vi "Decrypt with AES.vi"(0 "Password.In":string, 2 "BitKeyType(256)":u16(ring)=256 items=["AES bit key 128"=128, "AES bit key 192"=192, "AES bit key 256"=256], 7 "Encrypted Text In":string, 11 "error in":errorcluster) -> (8 "Decrypted Text Out":string, 15 "error out":errorcluster)   [LabVIEW 2012, in "Advanced Encryption Standard (AES).lvlib"]
doc: "Takes string encrypted with Advanced Encryption Standart (AES) and decrypts it into initial text. \n\nThis VI allows reentrant execution."
uses:
  Advanced Encryption Standard (AES).lvlib
  Controls and Typedefs/Decryption Phases Enum (Typedef).ctl
  Controls and Typedefs/Decipher Phases Enum (Typedef).ctl
panel:
  out "unsigned byte.utf8":u8[](array[numeric])
  out "unsigned byte.text":u8[](array[numeric])
  out "plaintxtByte":i32[](array[numeric])
  out "ciphertextArr":string[](array[string])
  out "ct":string[](array[string])
  out "nBlocks":i32
  out "cipherCntr":u16[](array[numeric])
  in  "0x100000000":u64=4294967296 format="%.0x"
  in  "blockSize":i32=16
  out "keySchedule":u32[](array[numeric])
  out "ctrTxt":string
  out "counterBlock":u32[](array[numeric])
  out "pwBytes":u32[](array[numeric])
  out "nBytes":i32
  # "Number of bits used in the key (256 by default).\nThe longer a key, the higher level of protection\nat expence of processor and RAM usage."
  # "Advanced Encryption Standart (AES)\nAES Decrypt 1.0"
  # "Receives Password in String format (plain text)"
  # "Receives encrypted text needed to be decrypted"
  # "Decrypted (plain) text"
  # "Development and Debugging"
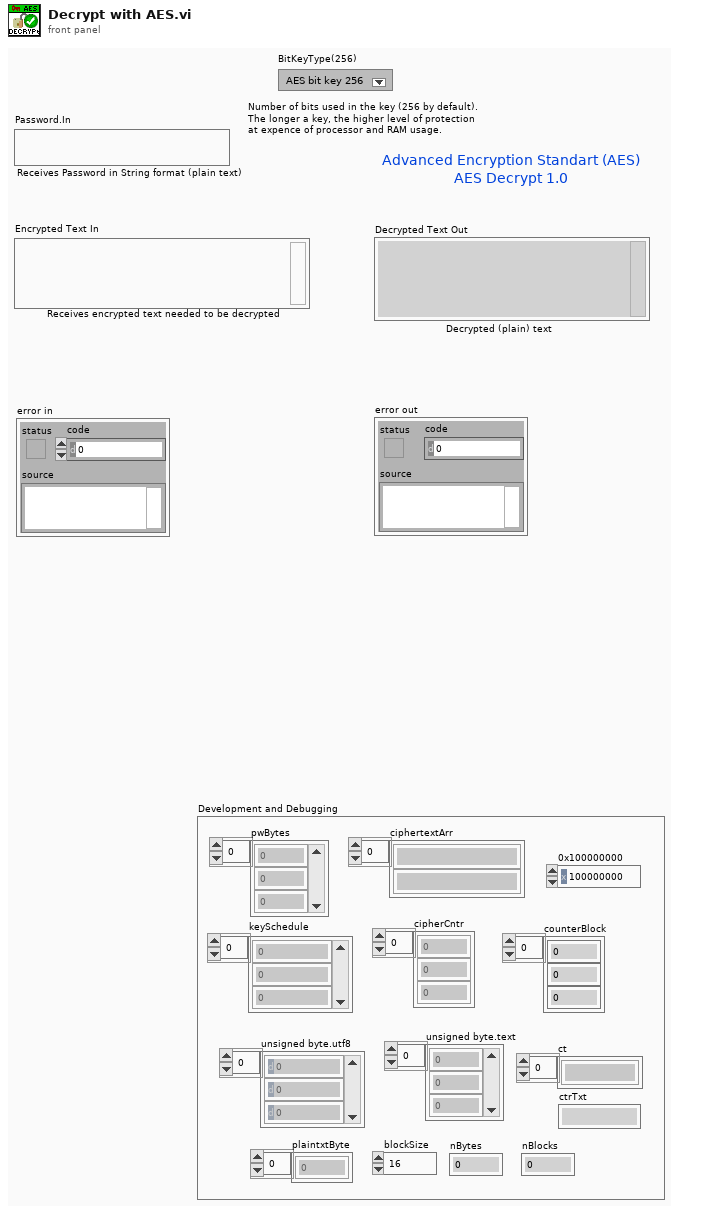
[diagram p1: front panel]
types:
  T1 = typedef "Decryption Phases Enum (Typedef).ctl" = enum16{"Init", "Decipher"}
  T2 = typedef "Decipher Phases Enum (Typedef).ctl" = enum16{"Logical Shifts", "Combine Bytes"}
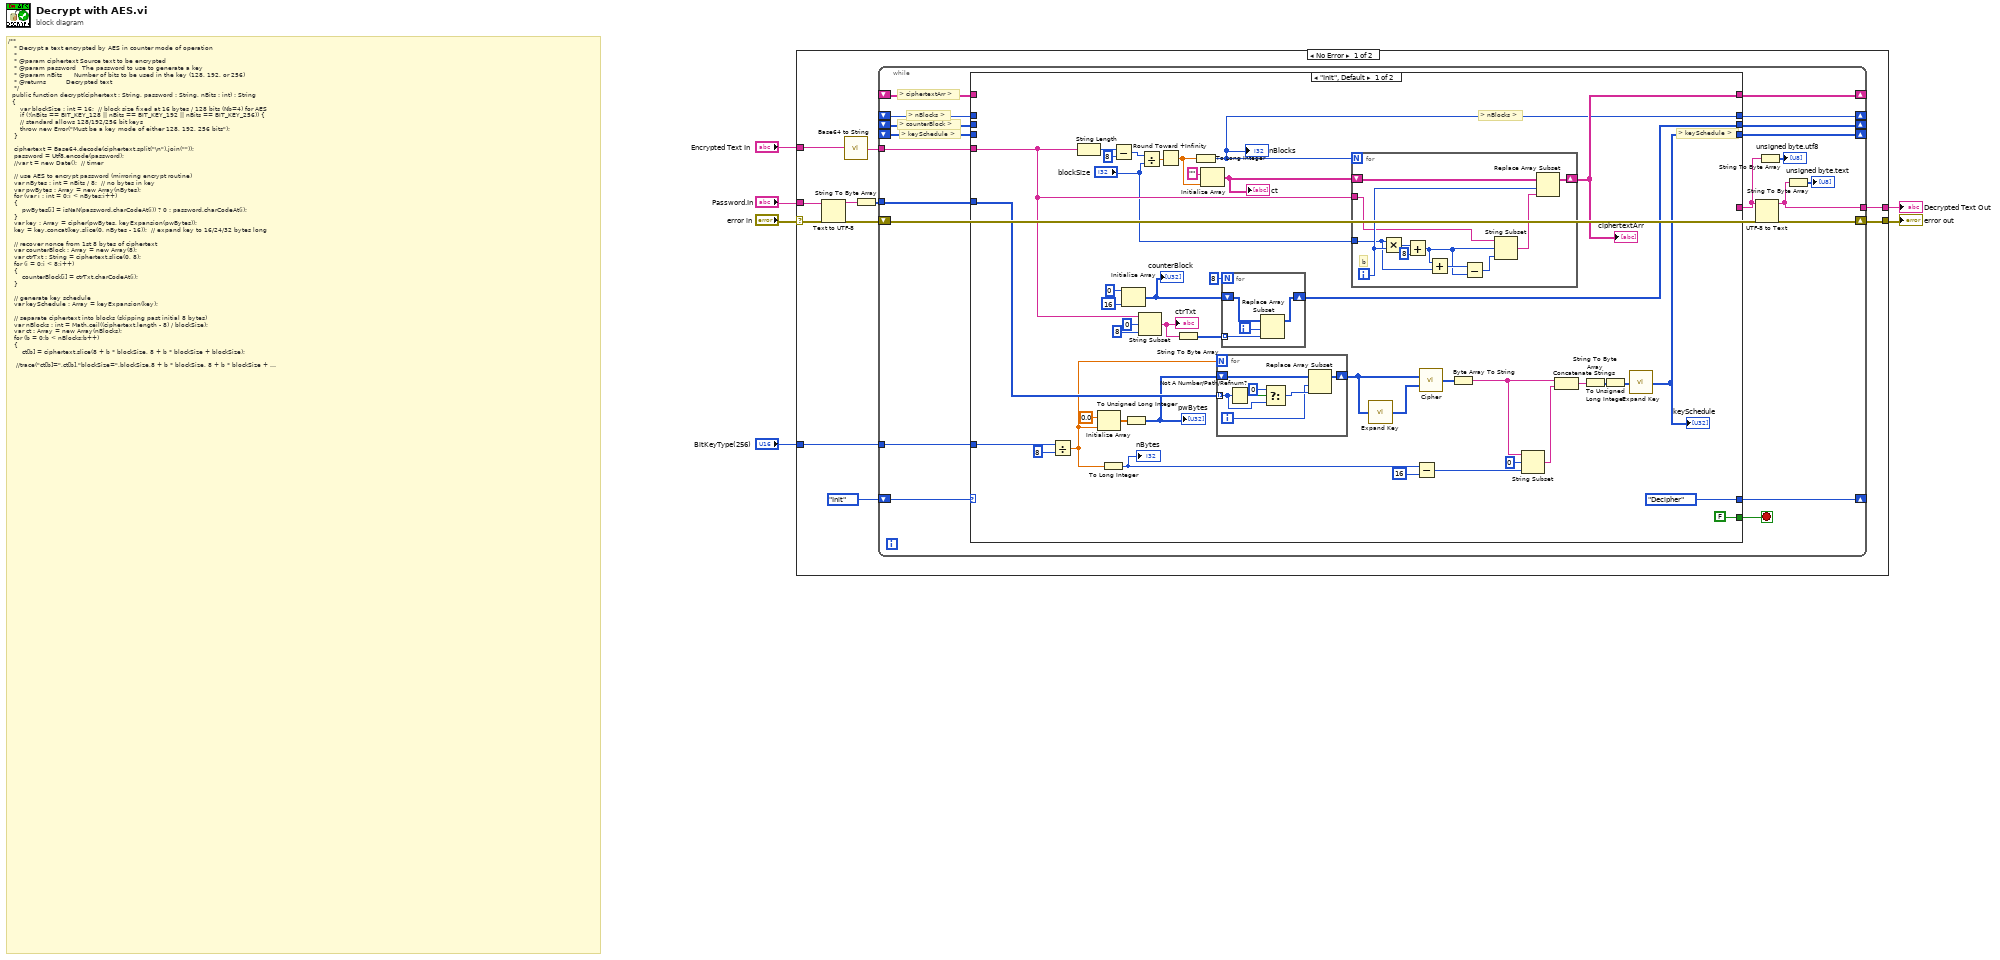
[diagram p0: block diagram]
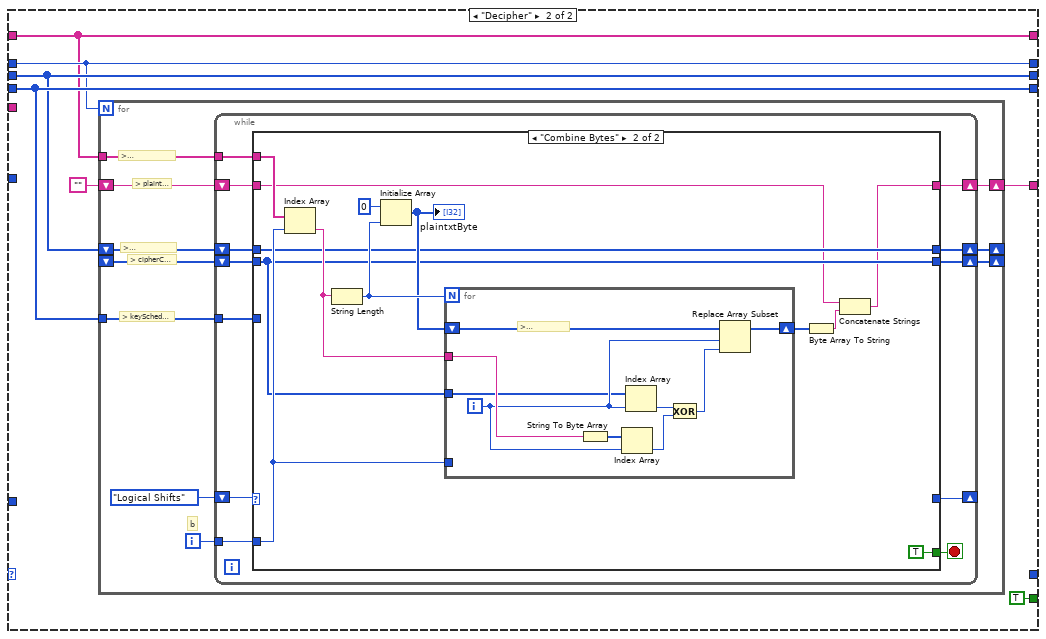
[diagram p2: hidden frame]
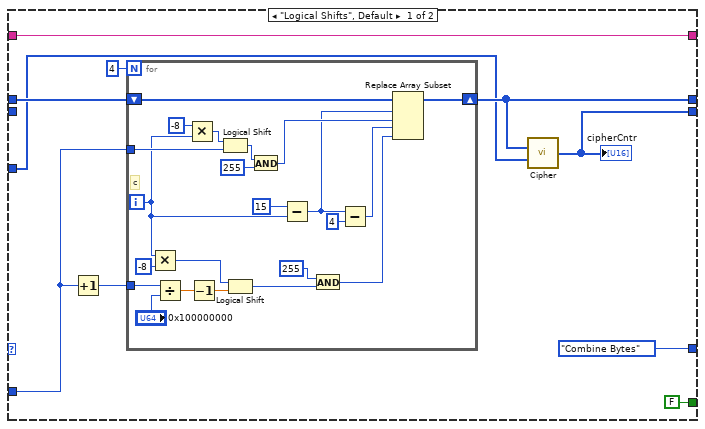
[diagram p3: hidden frame]
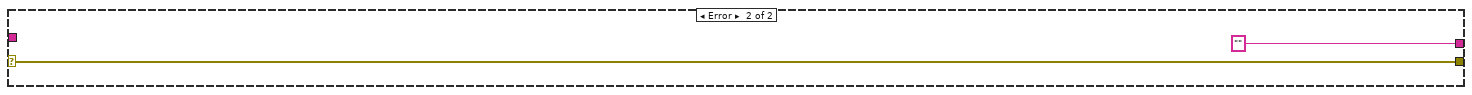
[diagram p4: hidden frame]
diagram:
  # "/** \n\t\t * Decrypt a text encrypted by AES in counter mode of operation\n\t\t *\n\t\t * @param ciphertext Source text to be encrypted\n\t\t * @param password   The password to use to generate a key\n\t\t * @param nBits      Number of bits to be used in the key (128, 192, or 256)\n\t\t * @returns          Decrypted text\n\t\t */\n\t\tpublic function decrypt(ciphertext : String, password : String, nBits : int) : String \n  {\n\t\t   \tvar blockSize : int = 16;  // block size fixed at 16 bytes / 128 bits (Nb=4) for AES\n\t\t   \tif (!(nBits == BIT_KEY_128 || nBits == BIT_KEY_192 || nBits == BIT_KEY_256)) {\n\t\t\t\t  // standard allows 128/192/256 bit keys\n\t\t\t\t  throw new Error(\"Must be a key mode of either 128, 192, 256 bits\");\n\t\t\t}\n\t\t\t\n\t\t\tciphertext = Base64.decode(ciphertext.split(\"\\n\").join(\"\"));\n\t\t\tpassword = Utf8.encode(password);\n\t\t\t//var t = new Date();  // timer\n\t\t\t  \n\t\t\t// use AES to encrypt password (mirroring encrypt routine)\n\t\t\tvar nBytes : int = nBits / 8;  // no bytes in key\n\t\t\tvar pwBytes : Array = new Array(nBytes);\n\t\t\tfor (var i : int = 0;i < nBytes;i++) \n\t\t\t{\n\t\t   \t\tpwBytes[i] = isNaN(password.charCodeAt(i)) ? 0 : password.charCodeAt(i);\n\t\t\t}\n\t\t\tvar key : Array = cipher(pwBytes, keyExpansion(pwBytes));\n\t\t\tkey = key.concat(key.slice(0, nBytes - 16));  // expand key to 16/24/32 bytes long\n\t\t\t\n\t\t\t// recover nonce from 1st 8 bytes of ciphertext\n\t\t\tvar counterBlock : Array = new Array(8);\n\t\t\tvar ctrTxt : String = ciphertext.slice(0, 8);\n\t\t\tfor (i = 0;i < 8;i++) \n\t\t\t{\n\t\t\t   \tcounterBlock[i] = ctrTxt.charCodeAt(i);\n\t\t\t}\n\t\t\t  \n\t\t\t// generate key schedule\n\t\t\tvar keySchedule : Array = keyExpansion(key);\n\t\t\t\n\t\t\t// separate ciphertext into blocks (skipping past initial 8 bytes)\n\t\t\tvar nBlocks : int = Math.ceil((ciphertext.length - 8) / blockSize);\n\t\t\tvar ct : Array = new Array(nBlocks);\n\t\t\tfor (b = 0;b < nBlocks;b++) \n\t\t\t{\n\t\t\t   \tct[b] = ciphertext.slice(8 + b * blockSize, 8 + b * blockSize + blockSize);\n\t\t\t\t\n\t\t\t\t//trace(\"ct[b]=\",ct[b],\"blockSize=\",blockSize,8 + b * blockSize, 8 + b * blockSize + blockSize);\n\t\t\t}\n\t\t\t//var temp:String=ct[1];\n//\t\t\tfor (var i:int=0;i<temp.length;i++)\n//\t\t\t{\n//\t\t\t\ttrace(\"ct[1]Byte Array:\",temp.charCodeAt(i));\n//\t\t\t}\n\t\t\t\n\t\t\tvar ciphertextArr : Array = ct;  // ciphertext is now array of block-length strings\n\t\t\t\n\t\t\t// plaintext will get generated block-by-block into array of block-length strings\n\t\t\tvar plaintxt : Array = new Array(ciphertextArr.length);\n\t\t\t\n\t\t\tfor (var b : int = 0;b < nBlocks;b++) \n\t\t\t{\n\t\t\t\t// set counter (block #) in last 8 bytes of counter block (leaving nonce in 1st 8 bytes)\n\t\t\t   \tfor (var c : int = 0;c < 4;c++) \n\t\t\t\t   {\n\t\t\t      \t\tcounterBlock[15 - c] = ((b) >>> c * 8) & 0xff;\n\t\t   \t\t}\n\t   \t\t\tfor (c = 0;c < 4;c++) \n\t  \t\t\t{\n\t\t     \t\t\tcounterBlock[15 - c - 4] = (((b + 1) / 0x100000000 - 1) >>> c * 8) & 0xff;\n\t\t\t  \t}\n\t\t\t\t//trace(counterBlock);\n\t\t\t\tvar cipherCntr : Array = cipher(counterBlock, keySchedule);  // encrypt counter block\n\t\t\t\t//trace(cipherCntr);\n\t\t\t\tvar plaintxtByte : Array = new Array(String(ciphertextArr[b]).length);\n\t\t\t\tfor (i = 0;i < String(ciphertextArr[b]).length;i++) \n\t\t\t\t{\n\t\t\t\t   \t// -- xor plaintxt with ciphered counter byte-by-byte --\n\t\t\t\t   \tplaintxtByte[i] = cipherCntr[i] ^ String(ciphertextArr[b]).charCodeAt(i);\n\t\t\t  \t\t//trace(\"i=\",i,\"plaintxtByte[i]=\",plaintxtByte[i],\"cipherCntr[i]=\",cipherCntr[i],\"String(ciphertextArr[b]).charCodeAt(i)=\",String(ciphertextArr[b]).charCodeAt(i));\n\t\t\t  \t\t//trace(plaintxtByte[i]);\n\t\t\t  \t\tplaintxtByte[i] = String.fromCharCode(plaintxtByte[i]);\n\t\t\t\t\t\n\t\t\t\t}\n\t\t\t\tplaintxt[b] = plaintxtByte.join('');\n\t\t\t}\n\t\t\t\n\t\t\t// join array of blocks into single plaintext string\n\t\t\tvar plaintext : String = plaintxt.join('');\n\t\t\tplaintext = Utf8.decode(plaintext);  // decode from UTF8 back to Unicode multi-byte chars\n\t\t\treturn plaintext;\n\t\t}"
  n1 = case shown="No Error" "error in" {
    selector: "error in" -> [w8 w186]
    tunnel: [w13 w186] -> w5
    tunnel: "Encrypted Text In" -> [w11 _]
    tunnel: "Password.In" -> [w10 _]
    tunnel: [w9 "" ("text")] -> w2
    tunnel: "BitKeyType(256)" -> [w7 _]
    frame No Error {
      n2 = Text to UTF-8(8:w8, 11:w10) -> (0:w12:errorcluster, 3:w16:string)
      n3 = call "Base64 to String.vi"("Base64 String"=w11) -> ("String"=w14:string)  [unwired: 13 in, 1 out]
      n4 = String To Byte Array(string=w16) -> (unsigned byte array=w15:u8[])
      n5 = while {
        shift-right: [w25] -> _
        shift-left: Decryption_Phases_Enum_(Typedef)."Init" ("Decrypt Phases") -> [w37]
        tunnel: w15 -> [w36]
        tunnel: w14 -> [w35]
        shift-right: [w33] -> _
        shift-left: _ -> [w32]
        shift-right: [w31] -> _
        shift-left: _ -> [w30]
        shift-right: [w29] -> _
        shift-left: _ -> [w28]
        shift-right: [w27] -> _
        shift-left: _ -> [w26]
        tunnel: [w21] -> w9
        shift-right: [w20] -> w13
        shift-left: w12 -> [w19]
        tunnel: w7 -> [w18]
        stop <- w34 stop-if-true
        # "> keySchedule >"
        # "> counterBlock >"
        # "> nBlocks >"
        # "> ciphertextArr >"
        n6 = case shown="\"Init\", Default" w37 {
          tunnel: w36 -> [w65 _]
          tunnel: w35 -> [w47 _]
          tunnel: [FALSE TRUE] -> w34
          tunnel: [w46 w104] -> w33
          tunnel: w32 -> [_ w104]
          tunnel: [w44 w105] -> w31
          tunnel: w30 -> [_ w105]
          tunnel: [w43 w106] -> w29
          tunnel: w28 -> [_ w106]
          tunnel: [w42 w108] -> w27
          tunnel: w26 -> [_ w108]
          tunnel: [Decryption_Phases_Enum_(Typedef)."Decipher" ("Decrypt Phases") _] -> w25
          tunnel: [_ w103] -> w22
          tunnel: w18 -> [w38 _]
          frame "Init", Default {
            # "> keySchedule >"
            # "> nBlocks >"
            n7 = Divide(x=w38, y=u16 8) -> (x/y=w52:dbl)
            n8 = String Length(string=w47) -> (length=w74:i32)
            n9 = Initialize Array(0.0 ("element"), w52) -> (w64:dbl[])
            n10 = To Long Integer(number=w52) -> (32bit integer=w51:i32)
            "nBytes" <- w51
            n11 = Subtract(x=w74, y=8) -> (x-y=w72:i32)
            n12 = Initialize Array(u32 0 ("y"), 16 ("dimension size")) -> (w62:u32[])
            "counterBlock" <- w62
            n13 = To Unsigned Long Integer(number=w64) -> (unsigned 32bit integer=w63:u32[])
            "pwBytes" <- w63
            n14 = String Subset(string=w47, offset (0)=0, length (rest)=8 ("length (rest)")) -> (substring=w68:string)
            "ctrTxt" <- w68
            n15 = Divide(x=w72, y="blockSize") -> (x/y=w71:dbl)
            n16 = Round Toward +Infinity(x=w71) -> (ceil(x): smallest int >= x=w50:dbl)
            n17 = String To Byte Array(string=w68) -> (unsigned byte array=w69:u8[])
            n18 = To Long Integer(number=w50) -> (32bit integer=w44:i32)
            "nBlocks" <- w44
            n19 = Initialize Array("", w50) -> (w49:string[])
            "ct" <- w49
            n20 = for {
              N: w52 -> [_]
              tunnel: w65 -> [w97] mode=indexing
              shift-right: [w95] -> w53
              shift-left: w63 -> [w96]
              i -> [w99]
              n21 = Not A Number/Path/Refnum?(number/path/refnum=w97) -> (NaN/Path/Refnum?=w101:bool)
              n22 = Select(t=0 ("f"), s=w101, f=w97) -> (s? t:f=w100:i32)
              n23 = Replace Array Subset(array=w96, new element=w100, index=w99) -> (w95:u32[])
            }
            n24 = for {
              N: 8 -> [_]
              tunnel: w69 -> [w94] mode=indexing
              shift-right: [w91] -> w43
              shift-left: w62 -> [w92]
              i -> [w93]
              n25 = Replace Array Subset(array=w92, new element=w94, index=w93) -> (w91:u32[])
            }
            n26 = for {
              N: w44 -> [_]
              shift-right: [w82] -> w46
              shift-left: w49 -> [w83]
              tunnel: w47 -> [w81]
              tunnel: "blockSize" -> [w80]
              i -> [w88]
              # "b"
              n27 = Multiply(x=w80, y=w88) -> (x*y=w90:i32)
              n28 = Add(x=w90, y=8) -> (x+y=w85:i32)
              n29 = Add(x=w85, y=w80) -> (x+y=w86:i32)
              n30 = Subtract(x=w86, y=w85) -> (x-y=w84:i32)
              n31 = String Subset(string=w81, offset (0)=w85, length (rest)=w84) -> (substring=w87:string)
              n32 = Replace Array Subset(array=w83, new element=w87, index=w88) -> (w82:string[])
            }
            "ciphertextArr" <- w46
            n33 = call "Expand Key.vi"("Key"=w53) -> ("Expanded Key"=w54:u32[])  [unwired: 13 in, 1 out]
            n34 = Subtract(x=w51, y=u8 16) -> (x-y=w59:i32)
            n35 = call "Cipher.vi"("Key(input)"=w53, "ExpandedKey(w)1D"=w54) -> ("Cypher Output"=w55:u16[])  [unwired: 12 in, 1 out]
            n36 = Byte Array To String(unsigned byte array=w55) -> (string=w56:string)
            n37 = String Subset(string=w56, offset (0)=0, length (rest)=w59) -> (substring=w60:string)
            n38 = Concatenate Strings(w56, w60) -> (w61:string)
            n39 = String To Byte Array(string=w61) -> (unsigned byte array=w41:u8[])
            n40 = To Unsigned Long Integer(number=w41) -> (unsigned 32bit integer=w40:u32[])
            n41 = call "Expand Key.vi"("Key"=w40) -> ("Expanded Key"=w42:u32[])  [unwired: 13 in, 1 out]
            "keySchedule" <- w42
          }
          frame "Decipher" {
            n42 = for {
              N: w105 -> [_]
              shift-right: [w116] -> _
              shift-left: w106 -> [w117]
              tunnel: w108 -> [w115]
              shift-right: [w114] -> _
              shift-left: _ -> [w113]
              tunnel: w104 -> [w112]
              shift-right: [w111] -> w103
              shift-left: "" -> [w110]
              i -> [w118]
              # "> keySchedule >"
              # "> ciphertextArr >"
              # "> plaintxt >"
              # "> cipherCntr >"
              # "> counterBlock >"
              # "b"
              n43 = while {
                tunnel: w118 -> [w130]
                shift-right: [w119] -> _
                shift-left: Decipher_Phases_Enum_(Typedef)."Logical Shifts" ("Decipher Phases") -> [w121]
                shift-right: [w128] -> w116
                shift-left: w117 -> [w129]
                tunnel: w115 -> [w127]
                shift-right: [w126] -> w114
                shift-left: w113 -> [w124]
                tunnel: w112 -> [w125]
                shift-right: [w123] -> w111
                shift-left: w110 -> [w122]
                stop <- w120 stop-if-true
                n44 = case shown="\"Combine Bytes\"" w121 {
                  tunnel: w130 -> [w138 w170]
                  tunnel: w129 -> [w137 w166]
                  tunnel: [w136 w166] -> w128
                  tunnel: w127 -> [w135 _]
                  tunnel: [w134 w167] -> w126
                  tunnel: w125 -> [_ w169]
                  tunnel: w124 -> [_ w167]
                  tunnel: [w133 w165] -> w123
                  tunnel: w122 -> [w133 w164]
                  tunnel: [FALSE TRUE] -> w120
                  tunnel: [Decipher_Phases_Enum_(Typedef)."Combine Bytes" ("Decipher Phases") _] -> w119
                  frame "Logical Shifts", Default {
                    n45 = Increment(x=w138) -> (x+1=w140:i32)
                    n46 = for {
                      N: 4 -> [_]
                      tunnel: w138 -> [w160]
                      tunnel: w140 -> [w154]
                      shift-right: [w141] -> w136
                      shift-left: w137 -> [w142]
                      i -> [w149]
                      # "c"
                      n47 = Multiply(x=w149, y=-8 ("x")) -> (x*y=w148:i32)
                      n48 = Divide(x=w154, y="0x100000000") -> (x/y=w151:dbl)
                      n49 = Multiply(x=-8, y=w149) -> (x*y=w153:i32)
                      n50 = Decrement(x=w151) -> (x-1=w147:dbl)
                      n51 = Logical Shift(y=w153, x=w160) -> (x << y=w162:i32)
                      n52 = Logical Shift(y=w148, x=w147) -> (x << y=w146:u32)
                      n53 = And(x=w162, y=u16 255 ("0xff")) -> (x .and. y?=w158:i32)
                      n54 = Subtract(x=15, y=w149) -> (x-y=w157:i32)
                      n55 = And(x=u16 255 ("0xff"), y=w146) -> (x .and. y?=w145:u32)
                      n56 = Subtract(x=w157, y=4) -> (x-y=w155:i32)
                      n57 = Replace Array Subset(array=w142, new element #1=w158, index #1=w157, new element #2=w145, index #2=w155) -> (w141:u32[])
                    }
                    n58 = call "Cipher.vi"("Key(input)"=w136, "ExpandedKey(w)1D"=w135) -> ("Cypher Output"=w134:u16[])  [unwired: 12 in, 1 out]
                    "cipherCntr" <- w134
                  }
                  frame "Combine Bytes" {
                    n59 = Index Array(array=w169, index=w170) -> (element=w172:string)
                    n60 = String Length(string=w172) -> (length=w173:i32)
                    n61 = Initialize Array(0, w173) -> (w168:i32[])
                    "plaintxtByte" <- w168
                    n62 = for {
                      N: w173 -> [_]
                      tunnel: w170 -> [_]
                      tunnel: w172 -> [w180]
                      shift-right: [w178] -> w175
                      shift-left: w168 -> [w177]
                      tunnel: w167 -> [w176]
                      i -> [w179]
                      # "> plaintxtByte >"
                      n63 = String To Byte Array(string=w180) -> (unsigned byte array=w183:u8[])
                      n64 = Index Array(array=w183, index=w179) -> (element=w182:u8)
                      n65 = Index Array(array=w176, index=w179) -> (element=w184:u16)
                      n66 = Exclusive Or(1:w182, 2:w184) -> (0:w181:u16)
                      n67 = Replace Array Subset(array=w177, new element=w181, index=w179) -> (w178:i32[])
                    }
                    n68 = Byte Array To String(unsigned byte array=w175) -> (string=w171:string)
                    n69 = Concatenate Strings(w164, w171) -> (w165:string)
                  }
                }
              }
            }
          }
        }
        n70 = UTF-8 to Text(8:w19, 11:w22) -> (0:w20:errorcluster, 3:w21:string)
        n71 = String To Byte Array(string=w22) -> (unsigned byte array=→"unsigned byte.utf8":u8[])
        n72 = String To Byte Array(string=w21) -> (unsigned byte array=→"unsigned byte.text":u8[])
      }
    }
    frame Error {
    }
  }
  "error out" <- w5
  "Decrypted Text Out" <- w2
